vi "Initialize.vi"(8 "error in (no error)":errorcluster, 10 "Instrument Configuration File":string, 11 "working_directory":string) -> (0 "error out":errorcluster)   [LabVIEW 2018]
uses:
  SesWrapper/SesWrapper.lvlib
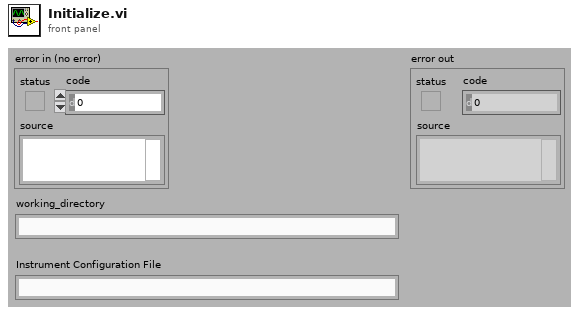
[diagram p1: front panel]
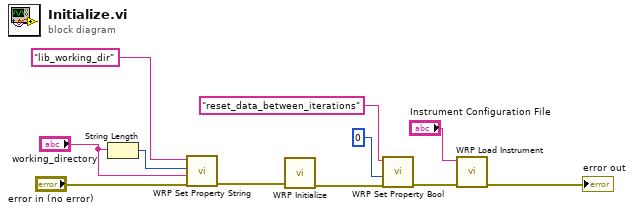
[diagram p0: block diagram]
diagram:
  n1 = String Length(string="working_directory") -> (length=w2:i32)
  n2 = call "WRP Set Property String.vi"("error in (no error)"="error in (no error)", "value"="working_directory", "index"=w2, "property"="lib_working_dir") -> ("error out"=w5:errorcluster)  [unwired: 6 in, 1 out]
  n3 = call "WRP Initialize.vi"("error in (no error)"=w5) -> ("error out"=w7:errorcluster)  [unwired: 8 in, 2 out]
  n4 = call "WRP Set Property Bool.vi"("error in (no error)"=w7, "value"=u8 0, "property"="reset_data_between_iterations") -> ("error out"=w10:errorcluster)  [unwired: 7 in, 1 out]
  n5 = call "WRP Load Instrument.vi"("error in (no error)"=w10, "fileName"="Instrument Configuration File") -> ("error out"=→"error out":errorcluster)  [unwired: 8 in, 1 out]
